vi "Filter.vi"(9 "time_const ms":dbl=1.0 min=1.0 max=3600000.0 format="%#_3g", 10 "PV":dbl format="%#_3g", 11 "Initialise":bool) -> (3 "PV_OUT":dbl format="%#_3g")   [LabVIEW 2019, in "Userlib.lvlib"]
uses:
  Userlib.lvlib
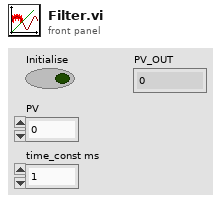
[diagram p1: front panel]
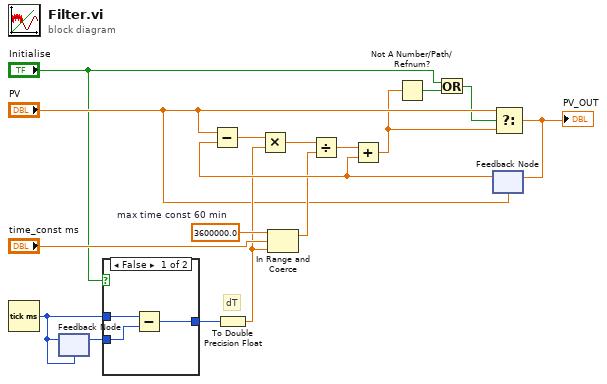
[diagram p0: block diagram]
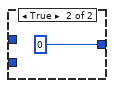
[diagram p2: hidden frame]
diagram:
  w12 = 3600000.0  # max time const 60 min
  # "dT"
  n1 = Tick Count (ms)() -> (millisecond timer value=w9:u32)
  n2 = feedback #1(w9) -> (w10:u32)
  n3 = feedback-in #1(w9) -> ()
  n4 = case shown="False" "Initialise" {
    tunnel: [w18 u32 0] -> w11
    tunnel: w10 -> [w19 _]
    tunnel: w9 -> [w20 _]
    frame False {
      n5 = Subtract(x=w20, y=w19) -> (x-y=w18:u32)
    }
    frame True {
    }
  }
  n6 = To Double Precision Float(number=w11) -> (double precision float=w8:dbl)
  n7 = In Range and Coerce(upper limit=w12, x="time_const ms", lower limit=w8) -> (coerced(x)=w14:dbl)  [unwired: 1 out]
  n8 = feedback #2("PV") -> (w15:dbl)
  n9 = Subtract(x="PV", y=w15) -> (x-y=w17:dbl)
  n10 = Multiply(x=w17, y=w8) -> (x*y=w16:dbl)
  n11 = Divide(x=w16, y=w14) -> (x/y=w7:dbl)
  n12 = Add(x=w7, y=w15) -> (x+y=w4:dbl)
  n13 = Not A Number/Path/Refnum?(number/path/refnum=w4) -> (NaN/Path/Refnum?=w3:bool)
  n14 = Or(x="Initialise", y=w3) -> (x .or. y?=w1:bool)
  n15 = Select(t="PV", s=w1, f=w4) -> (s? t:f=w5:dbl)
  "PV_OUT" <- w5
  n16 = feedback-in #2(w5) -> ()
